vi "ADIS16470 Open.vi"(8 "error in":errorcluster, 10 "Sychronous Process VI":T1, 11 "Hardware Config":T3={"SPI Clock Rate (Hz)"=1000000.0, "IMU SPI Mode (3)"=enum."Mode 3 (Clk Idle High,Sample on Trailing)", "IMU Reset Pin"=enum."SPI Port CS2", "IMU SPI Bus"=enum."SPI On-Board, CS0", "IMU Data Ready Pin"=enum."SPI Port CS1"}) -> (0 "error out":errorcluster, 3 "ADIS16470DevRef":T2={"DevStatus"={"status"=FALSE, "code"=0, "source"=""}, "Hardware Config"={"SPI Clock Rate (Hz)"=1000000.0, "IMU SPI Mode (3)"=enum."Mode 3 (Clk Idle High,Sample on Trailing)", "IMU Reset Pin"=enum."SPI Port CS2", "IMU SPI Bus"=enum."SPI On-Board, CS0", "IMU Data Ready Pin"=enum."SPI Port CS1"}, "End Calibration"=refnum, "Calibration Complete"=refnum, "Data FIFO"=refnum, "Status FIFO"=refnum, "Last Value Reference"=refnum, "Sychronous Process VI"=refnum})   [LabVIEW 2018]
uses:
  Typedef/ADIS16470 Hardware Configuration.ctl
  <vilib>/Rock Robotics/WPI/SPI/WPI_SPIMode.ctl
  <vilib>/Rock Robotics/SystemInterfaces/DIO/FPGA_DIOChannel.ctl
  <vilib>/Rock Robotics/SystemInterfaces/spilib/spi_bus.ctl
  Typedef/ADIS16470 Device Reference.ctl
  Typedef/ADIS16470 Data.ctl
  Typedef/ADIS16470 Status.ctl
  Typedef/ADIS16470 Process.ctl
  <vilib>/Rock Robotics/SystemInterfaces/NetworkCommunication/NetComm_UsageReport_ResourceType.ctl
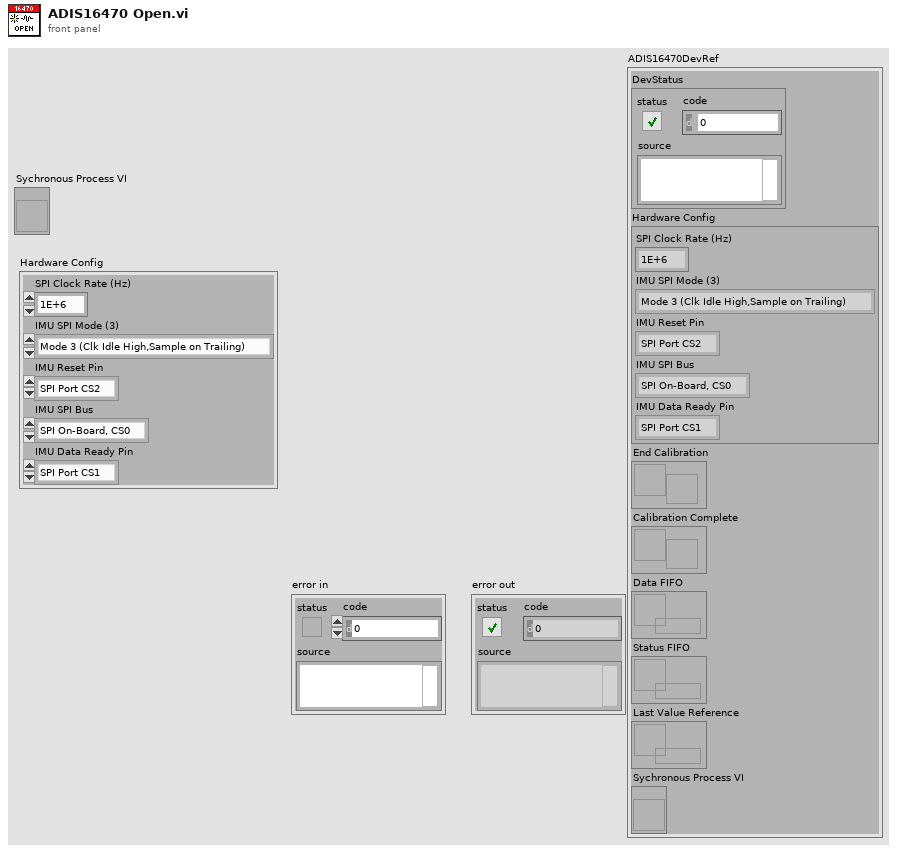
[diagram p1: front panel]
types:
  T1 = typedef "ADIS16470 Process.ctl" = refnum<vi>
  T2 = typedef "ADIS16470 Device Reference.ctl" = cluster{"DevStatus":errorcluster, "Hardware Config":T3, "End Calibration":refnum<notifier>, "Calibration Complete":refnum<notifier>, "Data FIFO":refnum<k33>, "Status FIFO":refnum<k33>, "Last Value Reference":refnum<data-value>, "Sychronous Process VI":T1}
  T3 = typedef "ADIS16470 Hardware Configuration.ctl" = cluster{"SPI Clock Rate (Hz)":dbl, "IMU SPI Mode (3)":T4, "IMU Reset Pin":T5, "IMU SPI Bus":T6, "IMU Data Ready Pin":T5}
  T4 = typedef "WPI_SPIMode.ctl" = enum16{"Mode 0 (Clk Idle Low,Sample on Leading)", "Mode 1 (Clk Idle Low,Sample on Trailing)", "Mode 2 (Clk Idle High,Sample on Leading)", "Mode 3 (Clk Idle High,Sample on Trailing)"}
  T5 = typedef "FPGA_DIOChannel.ctl" = enum8{"DIO 0", "DIO 1", "DIO 2", "DIO 3", "DIO 4", "DIO 5", "DIO 6", "DIO 7", "DIO 8", "DIO 9", "DIO MXP 0", "DIO MXP 1", "DIO MXP 2", "DIO MXP 3", "DIO MXP 4", "DIO MXP 5", "DIO MXP 6", "DIO MXP 7", "DIO MXP 8", "DIO MXP 9", "DIO MXP 10", "DIO MXP 11", "DIO MXP 12", "DIO MXP 13", "DIO MXP 14", "DIO MXP 15", "SPI Port CS1", "SPI Port CS2", "SPI Port CS3", "SPI Port MISO", "SPI Port MOSI", "Invalid"}
  T6 = typedef "spi_bus.ctl" = enum16{"SPI On-Board, CS0", "SPI On-Board, CS1", "SPI On-Board, CS2", "SPI On-Board, CS3", "SPI MXP", "Invalid"}
  T7 = typedef "ADIS16470 Data.ctl" = cluster{"Yaw":dbl, "Timestamp":dbl}
  T8 = typedef "ADIS16470 Status.ctl" = cluster{"Calibrated?":bool}
  T9 = typedef "NetComm_UsageReport_ResourceType.ctl" = enum8{"Controller", "Module", "Language", "CANPlugin", "Accelerometer", "ADXL345", "AnalogChannel", "AnalogTrigger", "AnalogTriggerOutput", "CANJaguar", "Compressor", "Counter", "Dashboard", "DigitalInput", "DigitalOutput", "DriverStationCIO", "DriverStationEIO", "DriverStationLCD", "Encoder", "GearTooth", "Gyro", "I2C", "Framework", "Jaguar", "Joystick", "Kinect", "KinectStick", "PIDController", "Preferences", "PWM", "Relay", "RobotDrive", "SerialPort", "Servo", "Solenoid", "SPI", "Task", "Ultrasonic", "Victor", "Button", "Command", "AxisCamera", "PCVideoServer", "SmartDashboard", "Talon", "HiTechnicColorSensor", "HiTechnicAccel", "HiTechnicCompass", "SRF08", "AnalogOutput", "Victor SP", "Talon SRX", "CAN Talon SRX", "ADXL362 Accel", "ADXRS450 Gyro", "Rev SPARK", "Mindsensors SD540", "Digital Filter", "ADIS16448", "PDP", "PCM", "PigeonIMU", "Nidec Brushless", "CTRE CANifier", "CTRE Future 0", "CTRE Future 1", "CTRE Future 2", "CTRE Future 3", "CTRE Future 4", "CTRE Future 5", "CTRE Future 6", "Linear Filter", "Xbox Controller", "USB Camera", "NavX", "Pixy", "Pixy2", "ScanseSweep", "Shuffleboard", "CAN", "Digilent DMC60", "PWM Victor SPX", "Rev SPARK MAX PWM", "Rev SPARK MAX CAN", "ADIS16470"}
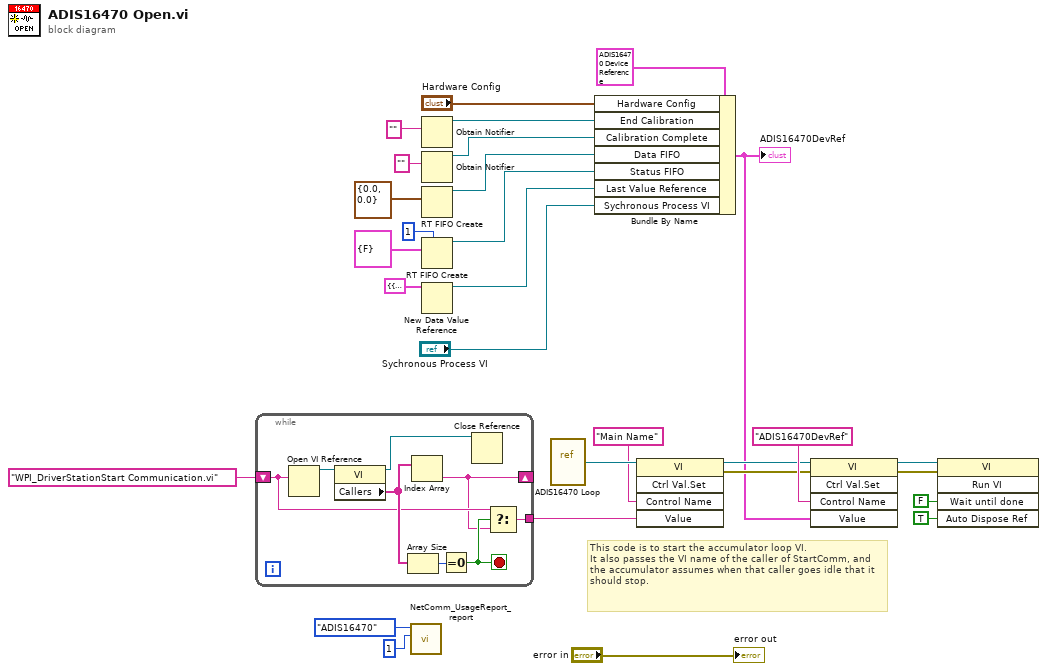
[diagram p0: block diagram]
diagram:
  # "This code is to start the accumulator loop VI.\nIt also passes the VI name of the caller of StartComm, and the accumulator assumes when that caller goes idle that it should stop."
  n1 = while {
    shift-right: [w32] -> _
    shift-left: "WPI_DriverStationStart Communication.vi" -> [w33]
    tunnel: [w31] -> w17
    stop <- w34 stop-if-true
    n2 = Open VI Reference(vi path=w33) -> (vi reference=w37:refnum<vi>)  [unwired: 1 in, 5 out]
    n3 = property class="VI"(reference=w37) -> (reference out=w30:refnum<vi>, "Callers"=w35:string[])  [unwired: 1 in, 1 out]
    n4 = Array Size(array=w35) -> (size(s)=w36:i32)
    n5 = Index Array(array=w35) -> (element=w32:string)  [unwired: 1 in]
    n6 = Equal To 0?(x=w36) -> (x = 0?=w34:bool)
    n7 = Close Reference(reference=w30) -> ()  [unwired: 1 in, 1 out]
    n8 = Select(t=w33, s=w34, f=w32) -> (s? t:f=w31:string)
  }
  n9 = call <vilib>:"NetComm_UsageReport_report.vi"("Instance Number"=u8 1, "Resource Type"=NetComm_UsageReport_ResourceType."ADIS16470") -> ()  [unwired: 10 in]
  n10 = Obtain Notifier(notification data type="") -> (notifier out=w11:refnum<notifier>)  [unwired: 3 in, 2 out]
  n11 = Obtain Notifier(notification data type="") -> (notifier out=w12:refnum<notifier>)  [unwired: 3 in, 2 out]
  n12 = RT FIFO Create(1:T7 {"Yaw"=0.0, "Timestamp"=0.0}) -> (8:w5:refnum<k33>)  [unwired: 7 in, 2 out]
  n13 = RT FIFO Create(1:T8 {"Calibrated?"=FALSE}, 4:u32 1 ("size (10)")) -> (8:w4:refnum<k33>)  [unwired: 6 in, 2 out]
  n14 = New Data Value Reference(data value=cluster{T7, T8} {{"Yaw"=0.0, "Timestamp"=0.0}, {"Calibrated?"=FALSE}} ("output cluster")) -> (data value reference=w2:refnum<data-value>)  [unwired: 1 in, 1 out]
  n15 = vi-ref "ADIS16470 Loop.vi"() -> (w19:refnum<vi>)
  n16 = Bundle By Name(cluster=T2 {"DevStatus"={"status"=FALSE, "code"=0, "source"=""}, "Hardware Config"={"SPI Clock Rate (Hz)"=1000000.0, "IMU SPI Mode (3)"=enum."Mode 3 (Clk Idle High,Sample on Trailing)", "IMU Reset Pin"=enum."SPI Port CS2", "IMU SPI Bus"=enum."SPI On-Board, CS0", "IMU Data Ready Pin"=enum."SPI Port CS1"}, "End Calibration"=refnum, "Calibration Complete"=refnum, "Data FIFO"=refnum, "Status FIFO"=refnum, "Last Value Reference"=refnum, "Sychronous Process VI"=refnum} ("ADIS16470DevRef"), "Hardware Config"="Hardware Config", "End Calibration"=w11, "Calibration Complete"=w12, "Data FIFO"=w5, "Status FIFO"=w4, "Last Value Reference"=w2, "Sychronous Process VI"="Sychronous Process VI") -> (w13:T2)
  "ADIS16470DevRef" <- w13
  n17 = invoke class="VI" method="Ctrl Val.Set"(reference=w19, "Control Name"="Main Name", "Value"=w17) -> (reference out=w16:refnum<vi>, error out=w21:errorcluster)  [unwired: 2 in, 3 out]
  n18 = invoke class="VI" method="Ctrl Val.Set"(reference=w16, error in=w21, "Control Name"="ADIS16470DevRef", "Value"=w13) -> (reference out=w26:refnum<vi>, error out=w22:errorcluster)  [unwired: 1 in, 3 out]
  n19 = invoke class="VI" method="Run VI"(reference=w26, error in=w22, "Wait until done"=FALSE ("Wait Until Done"), "Auto Dispose Ref"=TRUE ("Auto Dispose Reference")) -> ()  [unwired: 1 in, 5 out]
  "error out" <- "error in"
